vi "Meas_volt.vi"(8 "error in (no error)":errorcluster, 11 "Connection in":T1={"Baud"=9600, "Flow Ctl"=0, "COM port"="", "Parity"=0} {"Parity" items=["None", "Odd", "Even"]; "Flow Ctl" items=["None"]; "Baud" items=["4800"=4800, "9600"=9600, "19200"=19200, "38400"=38400]}) -> (0 "error out":errorcluster, 2 "Voltage":dbl, 3 "Connection out":T1={"Baud"=9600, "Flow Ctl"=0, "COM port"="", "Parity"=0} {"Parity" items=["None", "Odd", "Even"]; "Flow Ctl" items=["None"]; "Baud" items=["4800"=4800, "9600"=9600, "19200"=19200, "38400"=38400]})   [LabVIEW 2014, in "B&K Precision 9120 series.lvclass"]
uses:
  B&K Precision 9120 series.lvclass
  Serial_Config.ctl
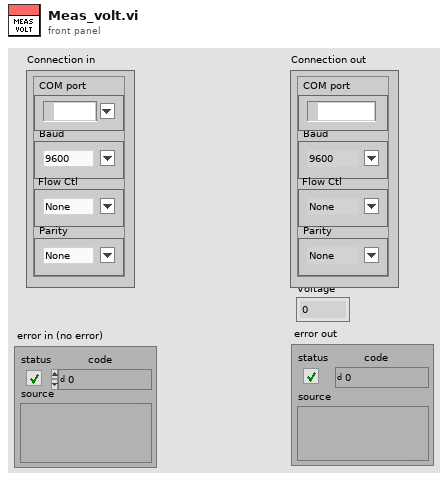
[diagram p1: front panel]
types:
  T1 = typedef "B&K Precision 9120 series.lvclass/Serial_Config.ctl" = cluster{"Baud":u32, "Flow Ctl":u16, "COM port":refnum<visa-resource-name>, "Parity":u16}
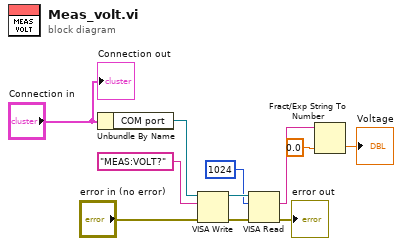
[diagram p0: block diagram]
diagram:
  n1 = Unbundle By Name("Connection in") -> ("COM port"=w2:refnum<visa-resource-name>)
  n2 = VISA Write(VISA resource name=w2, write buffer="MEAS:VOLT?", error in (no error)="error in (no error)") -> (VISA resource name out=w8:refnum<visa-resource-name>, error out=w10:errorcluster)  [unwired: 1 out]
  n3 = VISA Read(VISA resource name=w8, byte count=u32 1024, error in (no error)=w10) -> (read buffer=w3:string, error out=→"error out":errorcluster)  [unwired: 2 out]
  n4 = Fract/Exp String To Number(string=w3, default (0 dbl)=0.0 ("default (0 I32)")) -> (number=→"Voltage":dbl)  [unwired: 2 in, 1 out]
  "Connection out" <- "Connection in"
